vi "Determine Command type.vi"(10 "Destination_RT in":string, 11 "Soucer_RT in":string) -> (1 "command type out":enum16{"BCRT", "RTBC", "RTRT", "invalid"}(ring), 2 "Destination_RT out":string, 3 "Source_RT out":string)   [LabVIEW 2020, in "Configuration_Helper.lvlib"]
uses:
  Configuration_Helper.lvlib
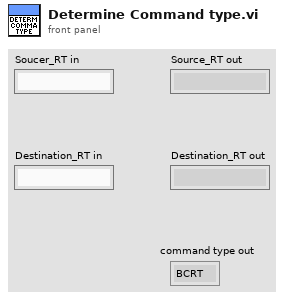
[diagram p1: front panel]
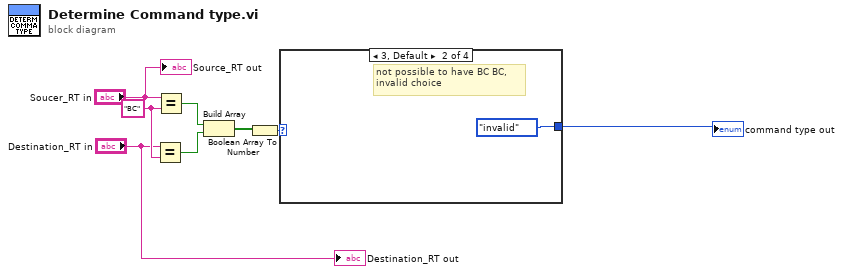
[diagram p0: block diagram]
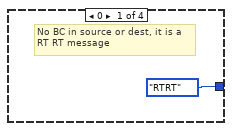
[diagram p2: hidden frame]
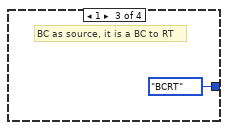
[diagram p3: hidden frame]
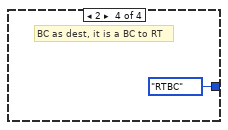
[diagram p4: hidden frame]
diagram:
  w6 = "BC" ("y")
  n1 = Equal?(x="Destination_RT in", y=w6) -> (x = y?=w7:bool)
  n2 = Equal?(x="Soucer_RT in", y=w6) -> (x = y?=w8:bool)
  n3 = Build Array(w8, w7) -> (w5:bool[])
  n4 = Boolean Array To Number(Boolean array=w5) -> (number=w4:u32)
  n5 = case shown="3, Default" w4 {
    tunnel: [enum16{"BCRT", "RTBC", "RTRT", "invalid"}."RTRT" ("command type out") enum16{"BCRT", "RTBC", "RTRT", "invalid"}."invalid" ("command type out") enum16{"BCRT", "RTBC", "RTRT"}."BCRT" ("command type out") enum16{"BCRT", "RTBC", "RTRT"}."RTBC" ("command type out")] -> w3
    frame 0 {
      # "No BC in source or dest, it is a\nRT RT message"
    }
    frame 3, Default {
      # "not possible to have BC BC, \ninvalid choice"
    }
    frame 1 {
      # "BC as source, it is a BC to RT"
    }
    frame 2 {
      # "BC as dest, it is a BC to RT"
    }
  }
  "command type out" <- w3
  "Destination_RT out" <- "Destination_RT in"
  "Source_RT out" <- "Soucer_RT in"
